vi "Spanwerte aufzeichnen.vi"(0 "Sollwerte":sgl, 2 "Komponente":u16(ring), 5 "Offset":sgl, 7 "Aktueller Spanfactor":sgl, 9 "Mittelung in sec":u32, 11 "error in (no error)":errorcluster caption="Fehler (Eingang, kein Fehler)") -> (3 "Aktuelle Fehler":sgl, 4 "Spanfaktor":sgl, 6 "Neuer Wert":sgl, 8 "Aktueller Wert gemittelt":sgl, 10 "Aktuelle Standardabweichung":sgl, 14 "neue Standardabweichung":sgl, 15 "error out":errorcluster caption="Fehler (Ausgang)")   [LabVIEW 2020, in "FT-IR.lvlib" / "Spanfaktor.lvlib"]
uses:
  Spanfaktor.lvlib
  FGV FT-IR Aktionen.ctl
  Messdaten/Aktionen FGV Messdaten.ctl
  Messdaten/Gewichtung (Stichprobe).ctl
  Messdaten/Messdaten.lvlib
  FT-IR.lvlib
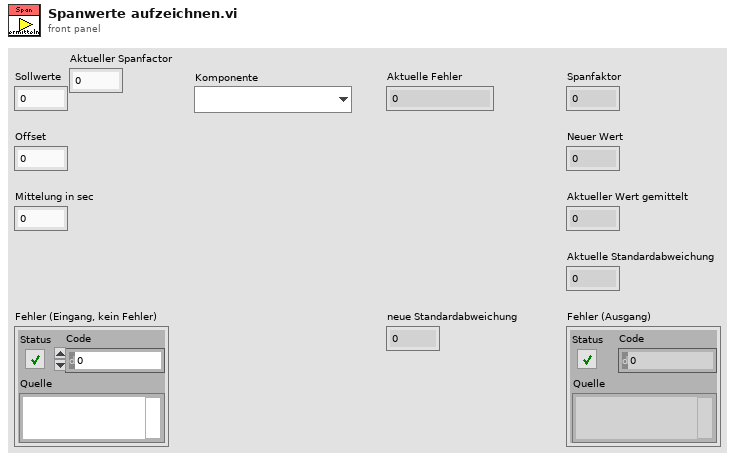
[diagram p1: front panel]
types:
  T1 = typedef "Messdaten.lvlib/Aktionen FGV Messdaten.ctl" = enum16{"lesen", "schreiben", "löschen", "Mittelwerte", "Komponente"}
  T2 = typedef "FT-IR.lvlib/FGV FT-IR Aktionen.ctl" = enum16{"lesen", "NOG setzen", "NOS setzen", "Initialisieren", "speichern", "ALLES setzen", "FT-IR Spektrum loggen", "Komm Stoppen", "Spektrum LogKonfig"}
  T3 = typedef "Messdaten.lvlib/Rolling Average Daten.ctl" = cluster{"RA aktuelle Messwerte":sgl[], "RA Messdaten":sgl[][], "RA Deviation":sgl[], "RA Zeitstempeln":timestamp[], "Rohwerte FTIR":sgl[][]}
  T4 = typedef "Messdaten.lvlib/Gewichtung (Stichprobe).ctl" = enum16{"Sample", "Population"}
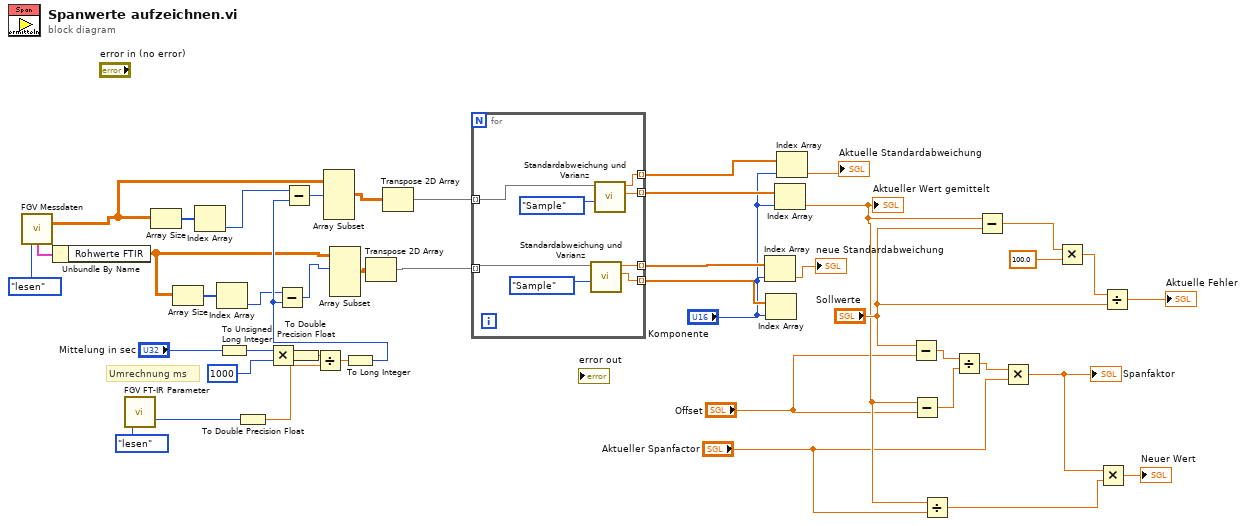
[diagram p0: block diagram]
diagram:
  # "Umrechnung ms"
  n1 = call "FGV Messdaten.vi"("Aktionen"=Aktionen_FGV_Messdaten."lesen") -> ("Messdaten"=w13:sgl[][], "Ausgangs-Cluster"=w20:T3)  [unwired: 6 in, 7 out]
  n2 = Unbundle By Name(w20) -> ("Rohwerte FTIR"=w8:sgl[][])
  n3 = call "FGV FT-IR Parameter.vi"("Aktion"=FGV_FT-IR_Aktionen."lesen") -> ("Zykluszeit Messdatenverteiler"=w22:u32)  [unwired: 11 in, 7 out]
  n4 = Array Size(array=w13) -> (size(s)=w16:i32[])
  n5 = Array Size(array=w8) -> (size(s)=w10:i32[])
  n6 = Index Array(array=w16) -> (element=w14:i32)  [unwired: 1 in]
  n7 = Index Array(array=w10) -> (element=w9:i32)  [unwired: 1 in]
  n8 = To Unsigned Long Integer(number="Mittelung in sec") -> (unsigned 32bit integer=w42:u32)
  n9 = To Double Precision Float(number=w22) -> (double precision float=w19:dbl)
  n10 = Multiply(x=w42, y=u32 1000) -> (x*y=w40:u32)
  n11 = To Double Precision Float(number=w40) -> (double precision float=w18:dbl)
  n12 = Divide(x=w18, y=w19) -> (x/y=w39:dbl)
  n13 = To Long Integer(number=w39) -> (32bit integer=w11:i32)
  n14 = Subtract(x=w9, y=w11) -> (x-y=w6:i32)
  n15 = Subtract(x=w14, y=w11) -> (x-y=w15:i32)
  n16 = Array Subset(array=w13, index (row)=w15) -> (w12:sgl[][])  [unwired: 3 in]
  n17 = Array Subset(array=w8, index (row)=w6) -> (w7:sgl[][])  [unwired: 3 in]
  n18 = Transpose 2D Array(2D array=w7) -> (transposed array=w44:sgl[][])
  n19 = Transpose 2D Array(2D array=w12) -> (transposed array=w36:sgl[][])
  n20 = for {
    tunnel: w44 -> [w47] mode=indexing
    tunnel: [w52] -> w28 mode=indexing
    tunnel: [w51] -> w38 mode=indexing
    tunnel: w36 -> [w46] mode=indexing
    tunnel: [w49] -> w35 mode=indexing
    tunnel: [w48] -> w30 mode=indexing
    n21 = call "Standardabweichung und Varianz.vi"("Gewichtung (Stichprobe)"=Gewichtung_(Stichprobe)."Sample", "X"=w47) -> ("Mittelwert"=w51:sgl, "Standardabweichung"=w52:sgl)  [unwired: 7 in, 1 out]
    n22 = call "Standardabweichung und Varianz.vi"("Gewichtung (Stichprobe)"=Gewichtung_(Stichprobe)."Sample", "X"=w46) -> ("Mittelwert"=w49:sgl, "Standardabweichung"=w48:sgl)  [unwired: 7 in, 1 out]
  }
  n23 = Index Array(array=w28, index="Komponente") -> (element=→"neue Standardabweichung":sgl)
  n24 = Index Array(array=w38, index="Komponente") -> ()  [unwired: 1 out]
  n25 = Index Array(array=w35, index="Komponente") -> (element=w4:sgl)
  "Aktueller Wert gemittelt" <- w4
  n26 = Index Array(array=w30, index="Komponente") -> (element=→"Aktuelle Standardabweichung":sgl)
  n27 = Subtract(x="Sollwerte", y="Offset") -> (x-y=w25:sgl)
  n28 = Subtract(x=w4, y="Offset") -> (x-y=w5:sgl)
  n29 = Divide(x=w4, y="Aktueller Spanfactor") -> (x/y=w1:sgl)
  n30 = Divide(x=w25, y=w5) -> (x/y=w24:sgl)
  n31 = Subtract(x=w4, y="Sollwerte") -> (x-y=w32:sgl)
  n32 = Multiply(x=w24, y="Aktueller Spanfactor") -> (x*y=w23:sgl)
  "Spanfaktor" <- w23
  n33 = Multiply(x=w32, y=sgl 100.0) -> (x*y=w34:sgl)
  n34 = Multiply(x=w23, y=w1) -> (x*y=→"Neuer Wert":sgl)
  n35 = Divide(x=w34, y="Sollwerte") -> (x/y=→"Aktuelle Fehler":sgl)
